vi "Builds Updated Callback.vi"(7 "Owner":refnum<class>, 11 "Builds":T1[](array[typedef])) -> ()   [LabVIEW 2020, in "PicoG-Processor.lvlib" / "GVIWebProcessorApp.lvclass"]
uses:
  GVIWebProcessorApp.lvclass
  WebProjectWatcher/Web Build.ctl
  GVIWebProcessorApp.lvclass/GVIWebProcessorApp.ctl
  WebProjectWatcher/WebProjectWatcher.lvclass
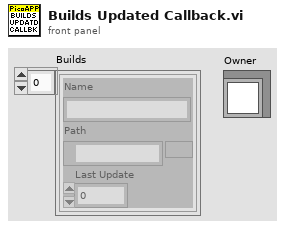
[diagram p1: front panel]
types:
  T1 = typedef "PicoG-Processor.lvlib/WebProjectWatcher.lvclass/Web Build.ctl" = cluster{"Name":string, "Path":path, "Last Update":dbl}
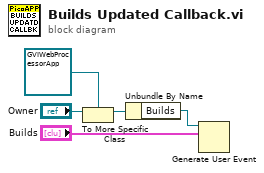
[diagram p0: block diagram]
diagram:
  n1 = To More Specific Class(target class=refnum<class "GVIWebProcessorApp.lvclass"> refnum ("PicoG-Processor:GVIWebProcessorApp.lvclass"), reference="Owner") -> (specific class reference=w3:refnum<class "GVIWebProcessorApp.lvclass">)  [unwired: 1 in, 1 out]
  n2 = Unbundle By Name(w3) -> ("Builds"=w2:refnum<user-event>)
  n3 = Generate User Event(user event=w2, event data cluster="Builds") -> ()  [unwired: 2 in, 2 out]
